vi "Create Path.vi"(8 "error in":errorcluster) -> (0 "error out":errorcluster, 3 "File Path Control":path)   [LabVIEW 2015, in "Logger.lvlib"]
uses:
  Logger.lvlib
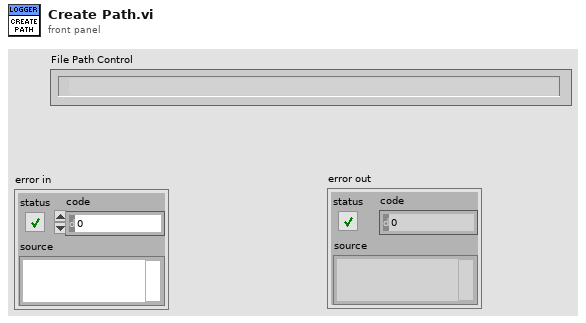
[diagram p1: front panel]
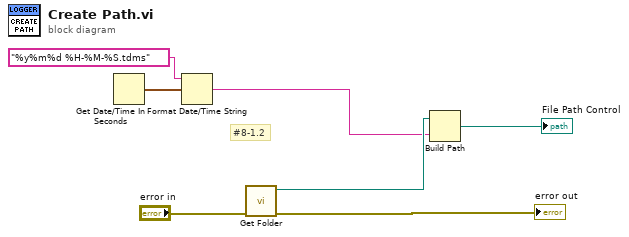
[diagram p0: block diagram]
diagram:
  # "#8-1.2"
  n1 = Get Date/Time In Seconds() -> (seconds since 1Jan1904=w3:timestamp)
  n2 = Format Date/Time String(time format string (%c)="%y%m%d %H-%M-%S.tdms", seconds (now)=w3) -> (date/time string=w1:string)  [unwired: 1 in]
  n3 = call "Get Folder.vi"("error in"="error in") -> ("error out"=→"error out":errorcluster, "dup path"=w6:path)  [unwired: 9 in]
  n4 = Build Path(base path=w6, name or relative path=w1) -> (appended path=→"File Path Control":path)
